vi "NPSV test.vi"() -> ()   [LabVIEW 2017]
uses:
  <vilib>/WPC Systems Ltd/GECO Driver/Lib/GECOMotion/GECOMotion/_typedefine/Axis Select.ctl
  <vilib>/WPC Systems Ltd/GECO Driver/Lib/GECOMotion/GECOMotion/GECO Motion.lvclass
  <vilib>/WPC Systems Ltd/GECO Driver/Lib/GECOBase/GECO_Driver Class/Motion/_typedefine/GECO_ActiveHighLow.ctl
  <vilib>/WPC Systems Ltd/GECO Driver/Lib/GECOBase/GECO_Driver Class/GECO_Driver.lvclass
  <vilib>/WPC Systems Ltd/GECO Driver/Lib/GECOBase/GECO_Driver Class/Motion/_typedefine/GECO_Motion Operation Mode.ctl
  GyroDef.ctl
  DataDef.ctl
  <vilib>/WPC Systems Ltd/GECO Driver/Lib/GECOBase/GECO_Driver Class/GECO_SlotName.ctl
  <vilib>/WPC Systems Ltd/GECO Driver/Lib/GECOBase/GECO_Driver Class/Motion/_typedefine/GECO_Stepper Output Configuration.ctl
  <vilib>/NI/Modbus Library/API/Modbus API.lvclass
  <vilib>/addons/control/pid/NI_PID_pid.lvlib
  <vilib>/addons/control/pid/pid.llb/PID (DBL).vi
  <vilib>/NI/Modbus Library/API/Wrapper/API Main.lvlib
  <vilib>/NI/Modbus Library/API/Wrapper/Create TCP Slave.vi
  <vilib>/WPC Systems Ltd/GECO Driver/GECODriver/GECO_Initialize_PC/Initialize VIs/Initialize_GECOUno_4HX.vi
  <vilib>/NI/Modbus Library/API/Slave/Modbus Slave.lvclass
  C:/Program Files (x86)/National Instruments/LabVIEW 2019/vi.lib/NI/Modbus Library/API/Modbus API.lvclass
panel:
  out "Axis 1":T1
  out "Axis 2":T1
  out "Axis 3":T1
  out "Program Period":u32
  in  "Main Setting Tab":T2(tab)
  in  "PID gains setting Tab":enum32{"Axis 1", "Axis 2", "Axis 3"}(tab)
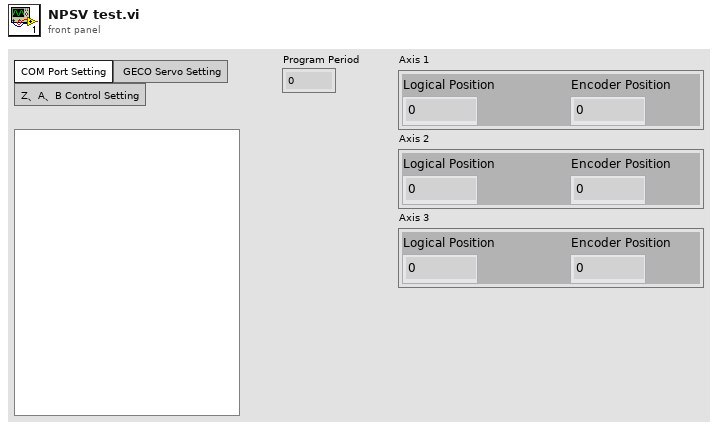
[diagram p1: front panel]
types:
  T1 = cluster{"Encoder Position":i32, "Logical Position":i32}
  T2 = enum32{"COM Port Setting", " GECO Servo Setting", "Z、A、B Control Setting"}
  T3 = typedef "DataDef.ctl" = cluster{"address starting":u16, "狀態":enum16{"初始化", "讀取", "寫入", "停止"}, "理想角度":cluster{"A":dbl, "B":dbl}, "register values":i16[], "Modbus COM":refnum<class "Modbus API.lvclass">, "TCP slave port":u16, " baud rate":u32, "Byte bits":u16, "ServoButtonControl":cluster{"三軸同退":bool, "三軸同進":bool, "三軸後退":bool, "三軸前進":bool, "二軸後退":bool, "二軸前進":bool, "一軸後退":bool, "一軸前進":bool}, "Serial Number":string, "GECO_Driver out":refnum<class "GECO_Driver.lvclass">, "number of inputs":u16, "ServoSetting":cluster{"Axis Select":T4, "Stepper Output Configuration":T5, "Motion Operation Mode":T6, "Motion Controller Slot":T7, "Singel Axis Move Paramters":cluster{"Motion Operation Mode":T6, "Target Position (0)":i32, "Velocity (10000)":i32, "Acceleration (100000)":u32, "Deacceleration (100000)":u32}, "Reverse":cluster{"Reverse Enable":bool, "Reverse Polarity":T8}, "Forward":cluster{"Forward Enable":bool, "Forward Polarity":T8}}, "GECO Motion out":refnum<class "GECO Motion.lvclass">, "Servo on":bool, "Axis 1 Position":cluster{"Encoder Position":i32, "Logical Position":i32}, "Axis 2 Position":cluster{"Encoder Position":i32, "Logical Position":i32}, "Axis 3 Position":cluster{"Encoder Position":i32, "Logical Position":i32}, "PIDSetting":cluster{"Z":i32, "A":i32, "B":i32, "Move Setting":T9, "Axis Pulse":dbl, "Axis Length":dbl, "PID gains ":cluster{"proportional gain (Kc)":dbl, "integral time (Ti, min)":dbl, "derivative time (Td, min)":dbl}}, "resource name":tag, "Save Path":refnum<file>}
  T4 = typedef "GECO Motion.lvclass/Axis Select.ctl" = enum16{"Axis 1", "Axis 2", "Axis 3", "Axis 4"}
  T5 = typedef "GECO_Driver.lvclass/GECO_Stepper Output Configuration.ctl" = enum16{"Step/Dir(One Pulse)", "CW/CCW(Two Pulse)"}
  T6 = typedef "GECO_Driver.lvclass/GECO_Motion Operation Mode.ctl" = enum16{"Absolute Position", "Relative Position", "Velocity"}
  T7 = typedef "GECO_Driver.lvclass/GECO_SlotName.ctl" = enum16{"C1", "C2", "C3", "C4"}
  T8 = typedef "GECO_Driver.lvclass/GECO_ActiveHighLow.ctl" = enum16{"Active High", "Active Low"}
  T9 = typedef "­y¸ñ.ctl" = u16
  T10 = typedef "GyroDef.ctl" = cluster{"Byte bits":u16, "baud rate":u32, "實際角度":cluster{"A":dbl, "B":dbl}, "COM Port":refnum<visa-resource-name>, "Save Path":refnum<file>}
  T11 = cluster{"Motion Operation Mode":T6, "Target Position (0)":i32, "Velocity (10000)":i32, "Acceleration (100000)":u32, "Deacceleration (100000)":u32}
  T12 = cluster{"Forward Enable":bool, "Forward Polarity":T8}
  T13 = cluster{"Reverse Enable":bool, "Reverse Polarity":T8}
  T14 = cluster{"三軸同退":bool, "三軸同進":bool, "三軸後退":bool, "三軸前進":bool, "二軸後退":bool, "二軸前進":bool, "一軸後退":bool, "一軸前進":bool, "Reset Encoder Position":bool, "AlarmReset":bool}[]
  T15 = cluster{"三軸同退":bool, "三軸同進":bool, "三軸後退":bool, "三軸前進":bool, "二軸後退":bool, "二軸前進":bool, "一軸後退":bool, "一軸前進":bool, "Reset Encoder Position":bool, "AlarmReset":bool}
  T16 = enum16{"open", "replace", "create", "open or create", "replace or create", "replace or create with confirmation"}
  T17 = cluster{"Logical Position":i32, "Encoder Position":i32}
  T18 = enum16{"Step/Dir(One Pulse)", "CW/CCW(Two Pulse)"}
  T19 = enum16{"Absolute Position", "Relative Position", "Velocity"}
  T20 = cluster{"proportional gain (Kc)":dbl, "integral time (Ti, min)":dbl, "derivative time (Td, min)":dbl}
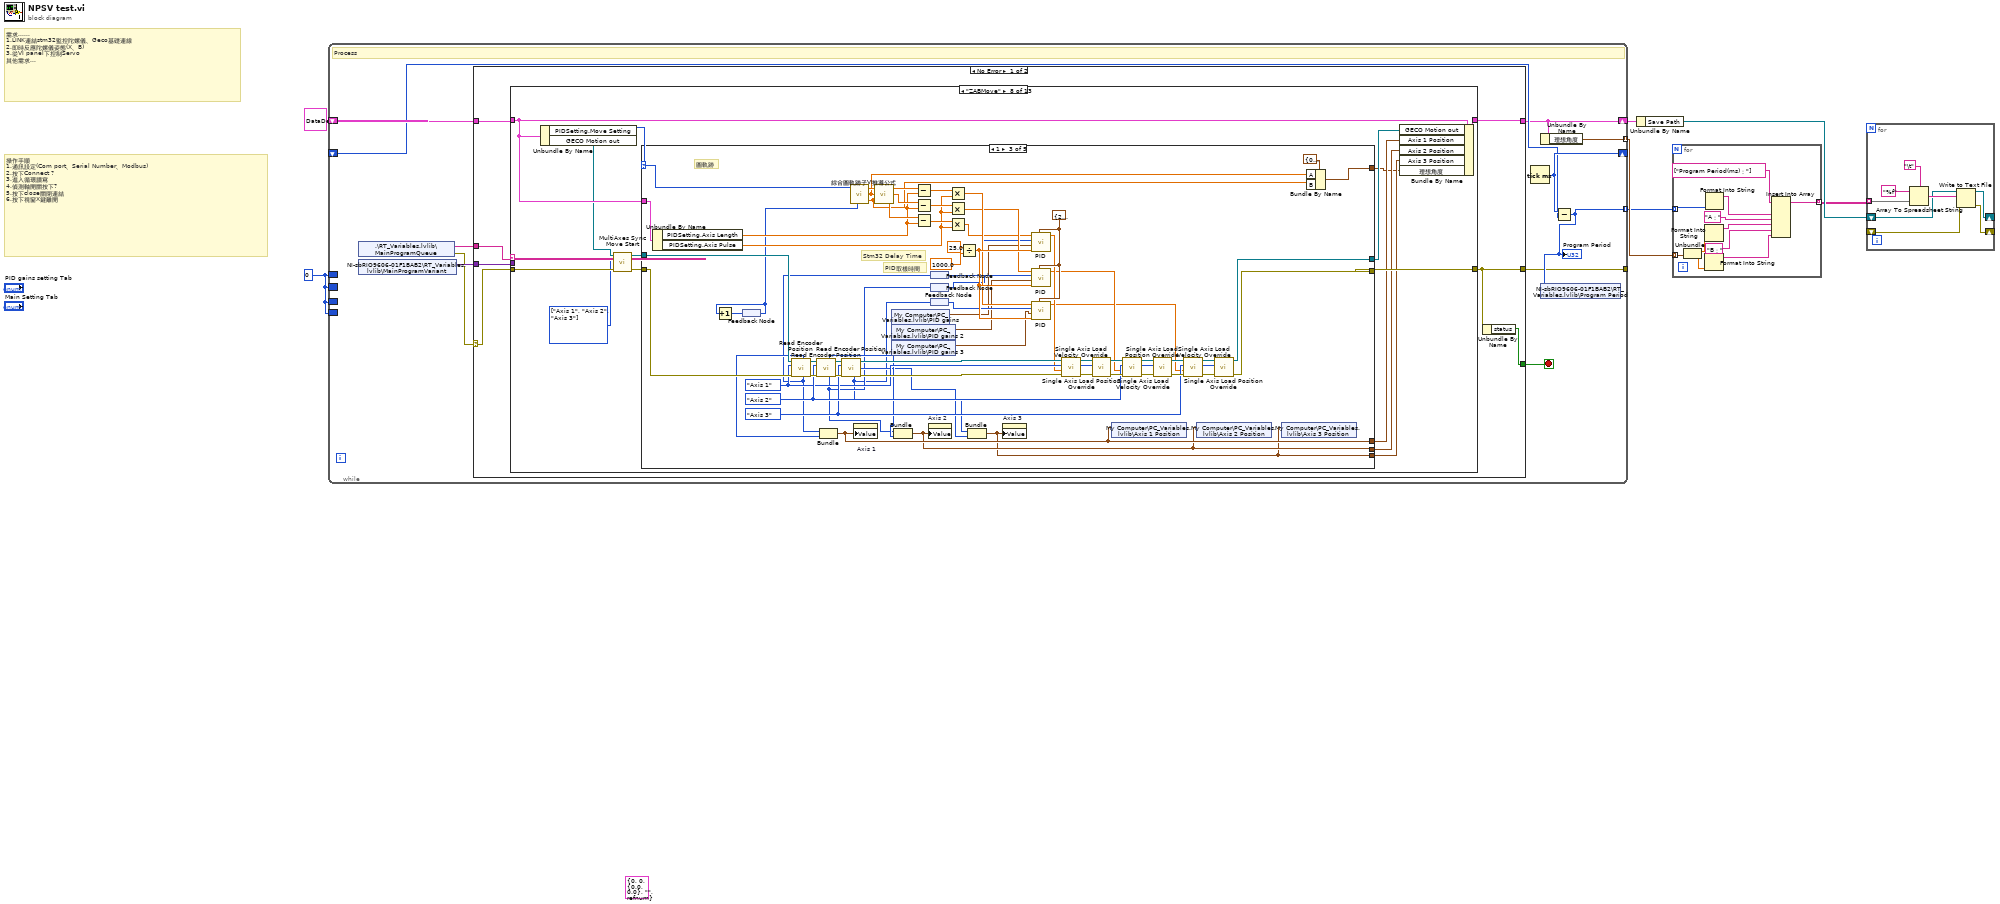
[diagram p0: block diagram]
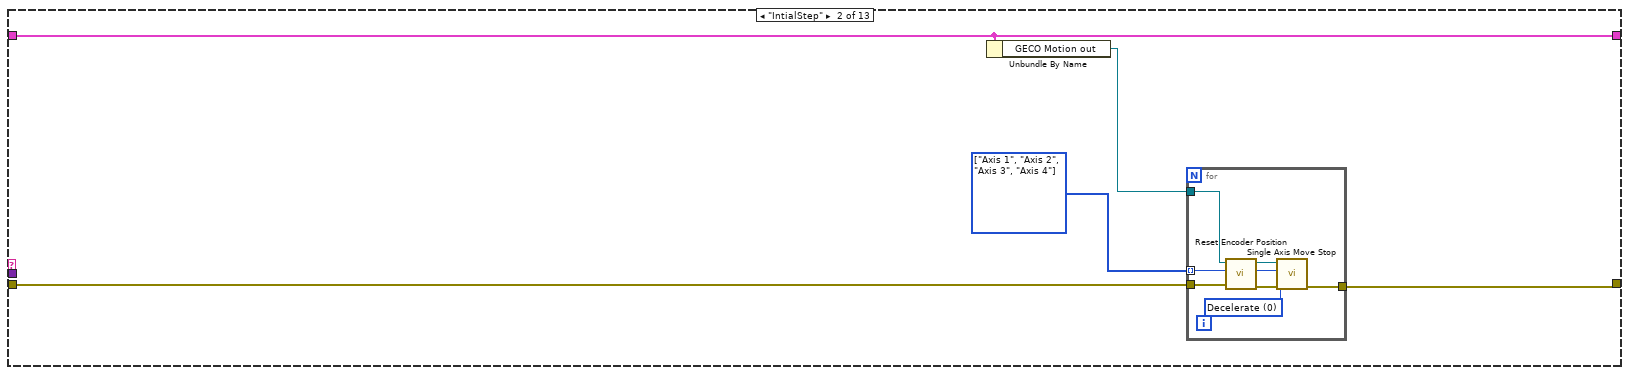
[diagram p3: hidden frame]
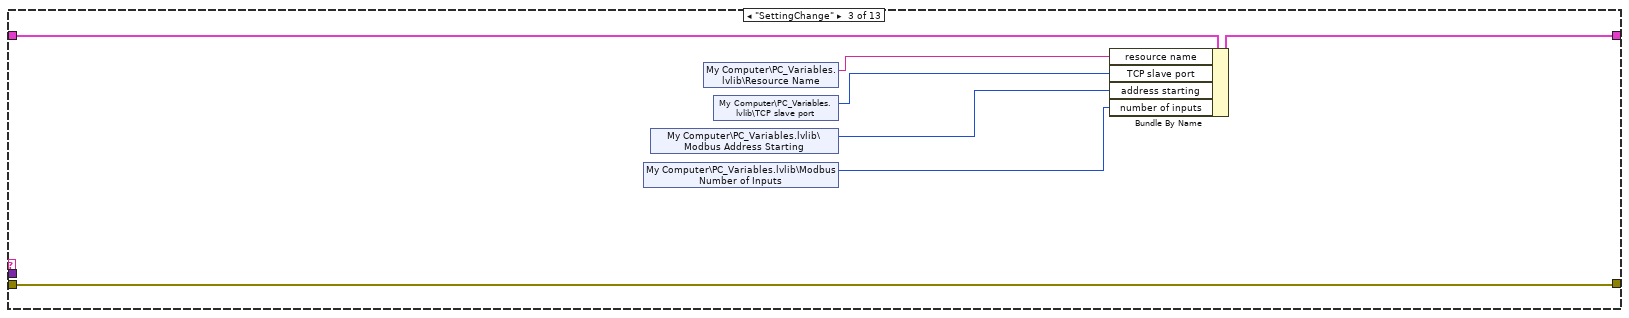
[diagram p4: hidden frame]
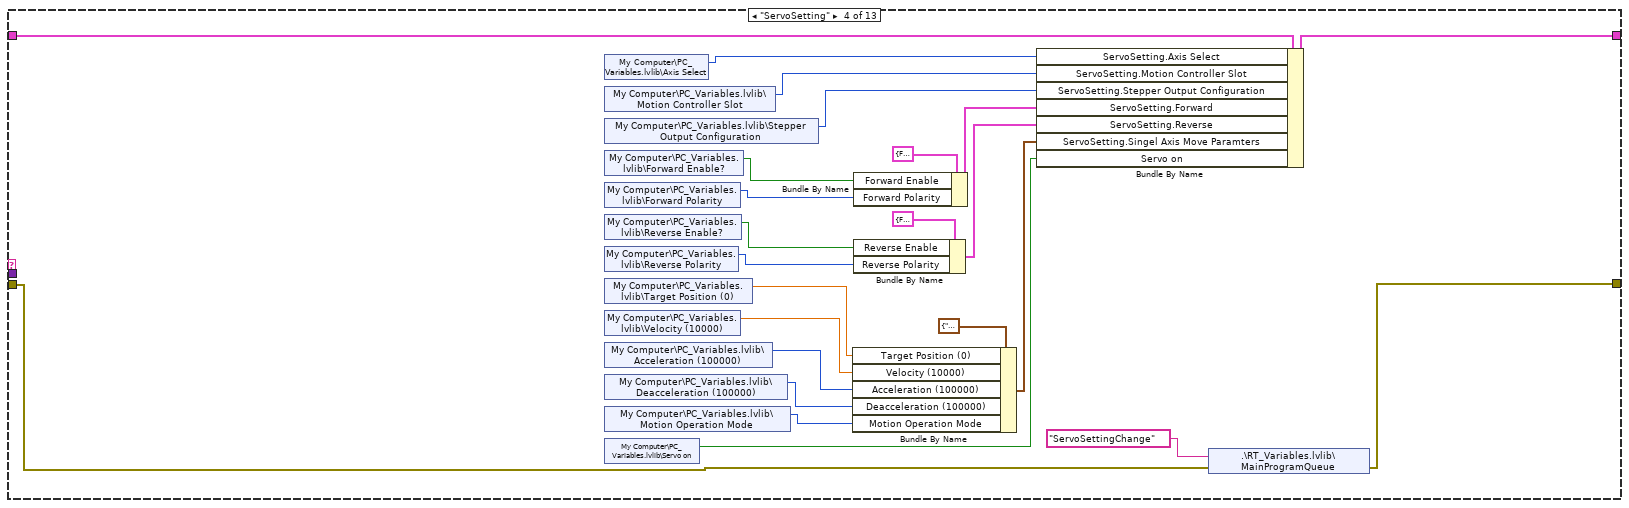
[diagram p5: hidden frame]
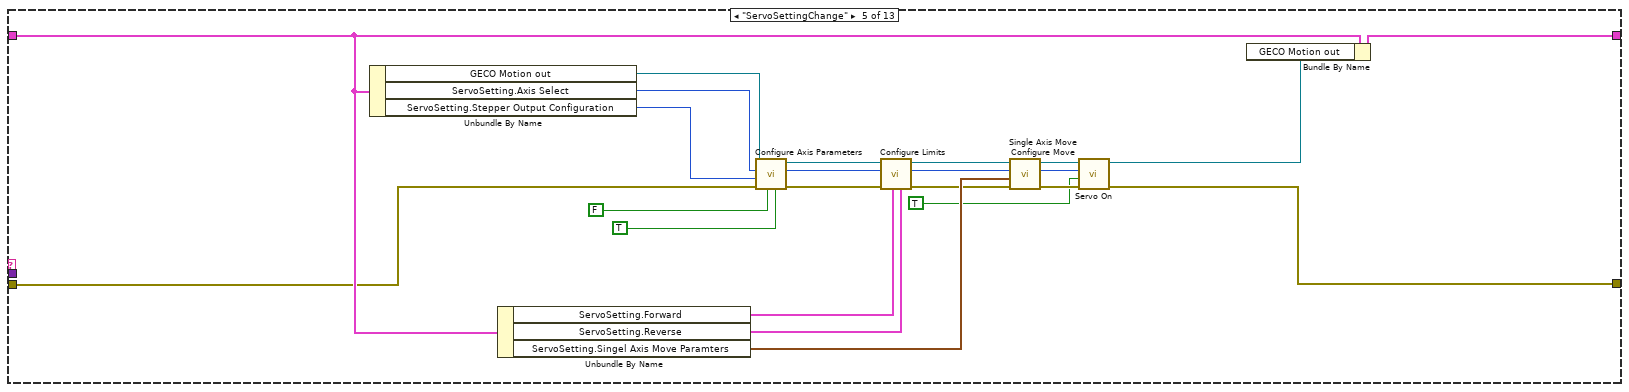
[diagram p6: hidden frame]
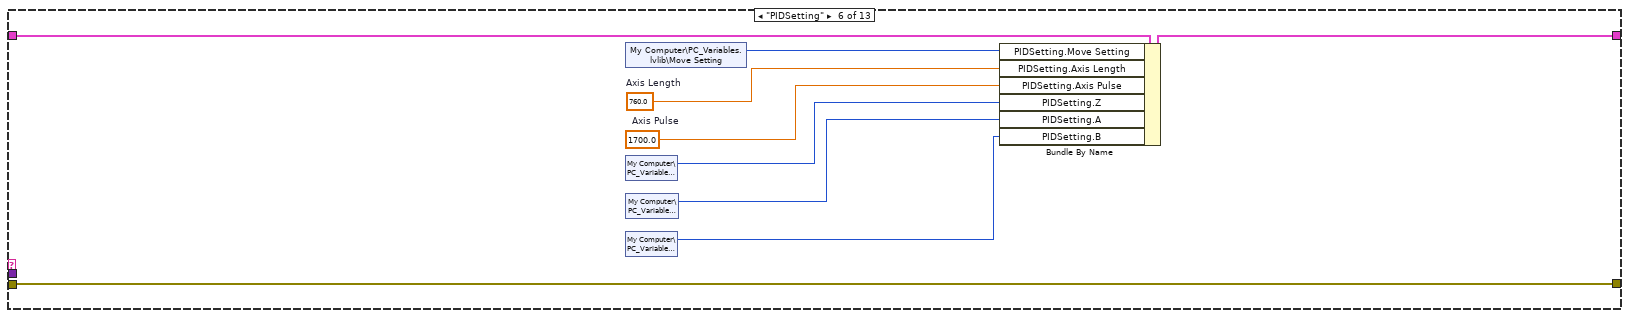
[diagram p7: hidden frame]
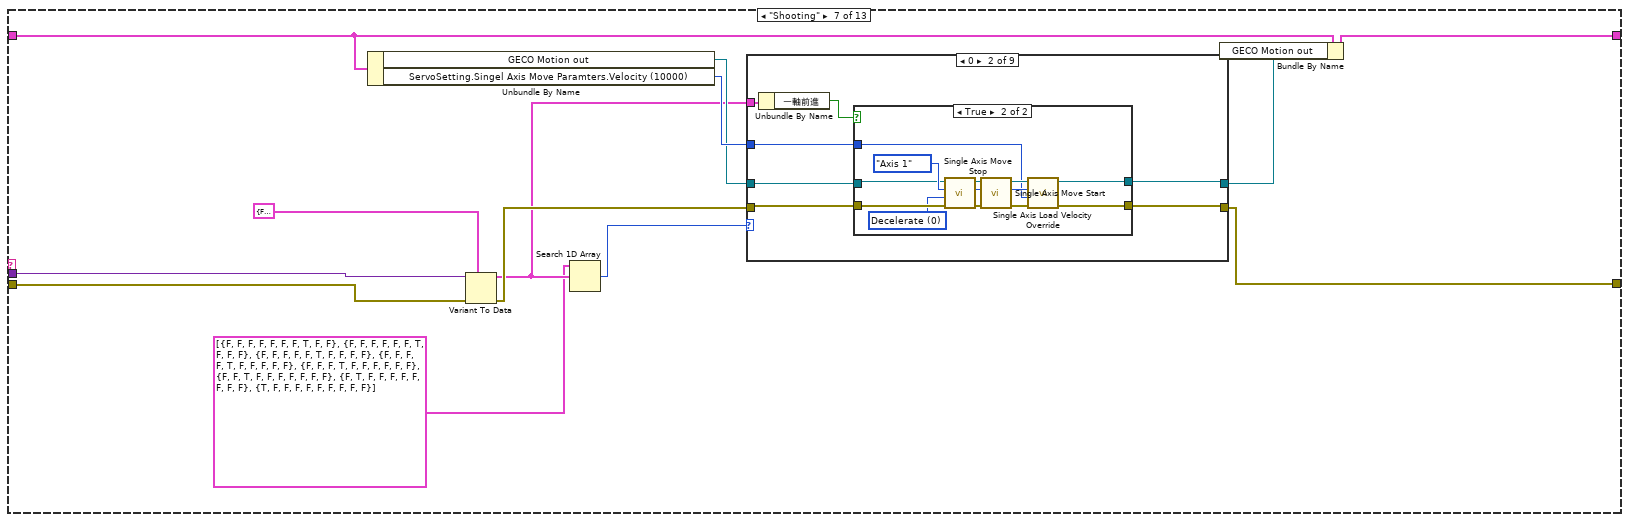
[diagram p8: hidden frame]
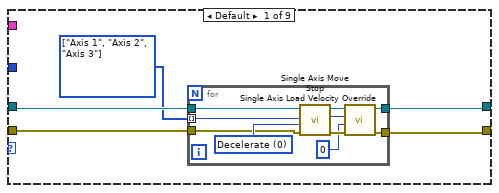
[diagram p9: hidden frame]
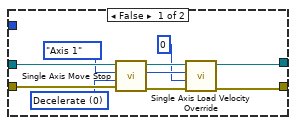
[diagram p10: hidden frame]
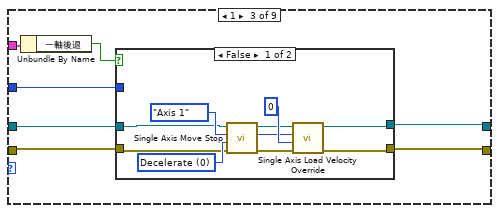
[diagram p11: hidden frame]
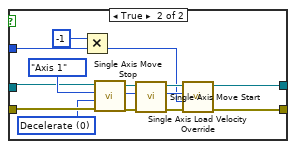
[diagram p12: hidden frame]
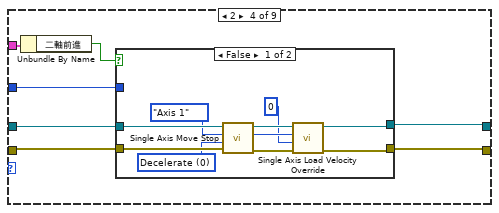
[diagram p13: hidden frame]
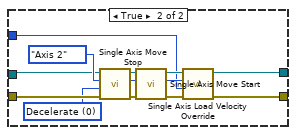
[diagram p14: hidden frame]
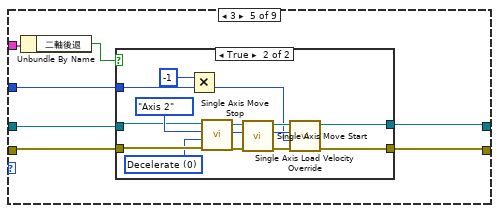
[diagram p15: hidden frame]
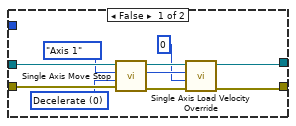
[diagram p16: hidden frame]
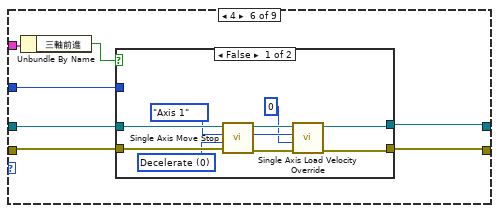
[diagram p17: hidden frame]
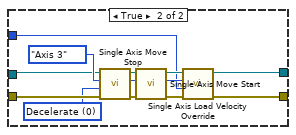
[diagram p18: hidden frame]
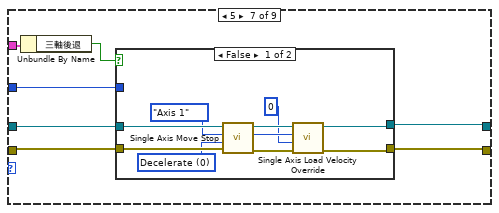
[diagram p19: hidden frame]
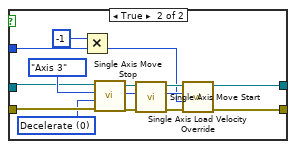
[diagram p20: hidden frame]
diagram:
  w6 = 0
  (unwired) T10 {"Byte bits"=0, "baud rate"=0, "實際角度"={"A"=0.0, "B"=0.0}, "COM Port"="", "Save Path"=refnum}
  # "操作手順\n1.通訊設定(Com port、Serial Number、Modbus)\n2.按下Connect ?\n3.進入循環讀寫\n4.偵測軸開關按下?\n5.按下close關閉連結\n6.按下視窗X鍵離開"
  # "需求......\n1.LINK連結stm32監控陀螺儀、Geco基礎連線\n2.即時反應陀螺儀姿態(X、B)\n3.從VI panel下控制Servo\n其他需求..."
  n1 = while {
    shift-right: [w14] -> w3
    shift-left: T3 {"address starting"=0, "狀態"=enum."初始化", "理想角度"={"A"=0.0, "B"=0.0}, "register values"=[], "Modbus COM"=refnum, "TCP slave port"=1, " baud rate"=0, "Byte bits"=0, "ServoButtonControl"={"三軸同退"=FALSE, "三軸同進"=FALSE, "三軸後退"=FALSE, "三軸前進"=FALSE, "二軸後退"=FALSE, "二軸前進"=FALSE, "一軸後退"=FALSE, "一軸前進"=FALSE}, "Serial Number"="", "GECO_Driver out"=refnum, "number of inputs"=0, "ServoSetting"={"Axis Select"=enum."Axis 1", "Stepper Output Configuration"=enum."Step/Dir(One Pulse)", "Motion Operation Mode"=enum."Absolute Position", "Motion Controller Slot"=enum."C1", "Singel Axis Move Paramters"={"Motion Operation Mode"=enum."Velocity", "Target Position (0)"=10000, "Velocity (10000)"=1, "Acceleration (100000)"=100000, "Deacceleration (100000)"=1}, "Reverse"={"Reverse Enable"=FALSE, "Reverse Polarity"=enum."Active Low"}, "Forward"={"Forward Enable"=FALSE, "Forward Polarity"=enum."Active Low"}}, "GECO Motion out"=refnum, "Servo on"=FALSE, "Axis 1 Position"={"Encoder Position"=0, "Logical Position"=0}, "Axis 2 Position"={"Encoder Position"=0, "Logical Position"=0}, "Axis 3 Position"={"Encoder Position"=0, "Logical Position"=0}, "PIDSetting"={"Z"=10000, "A"=10000, "B"=10000, "Move Setting"=1, "Axis Pulse"=10000.0, "Axis Length"=10000.0, "PID gains "={"proportional gain (Kc)"=1.0, "integral time (Ti, min)"=0.01, "derivative time (Td, min)"=0.0}}, "resource name"="", "Save Path"=refnum} -> [w17]
    shift-right: [w16] -> _
    shift-left: _ -> [w15]
    border: w6 -> [_]
    border: w6 -> [_]
    border: w6 -> [_]
    border: w6 -> [_]
    tunnel: [w13] -> w5 mode=indexing
    tunnel: [w12] -> w4 mode=indexing
    tunnel: [w11] -> _
    stop <- w18 stop-if-true
    # "Process"
    n2 = shared-variable ".\\RT_Variables.lvlib\\MainProgramQueue"() -> (w9:string, error out=w8:errorcluster)  [unwired: 1 in]
    n3 = shared-variable "NI-sbRIO9606-01F1BAB2\\RT_Variables.lvlib\\MainProgramVariant"() -> (w10:variant)  [unwired: 1 in, 1 out]
    n4 = case shown="No Error" w8 {
      selector: w8 -> [w23 w629]
      tunnel: [w22 TRUE] -> w18
      tunnel: [w25 w630] -> w14
      tunnel: w17 -> [w24 w630]
      tunnel: [w21 w629] -> w11
      tunnel: w10 -> [w20 _]
      tunnel: w9 -> [w19 _]
      frame No Error {
        n5 = case shown="\"ZABMove\"" w19 {
          tunnel: [w27 w29 w46 w70 w94 w102 w114 w404 w538 w554 w587 w609 w620] -> w25
          tunnel: w24 -> [w27 w29 w47 w71 w93 w103 w108 w406 w541 w557 w588 w611 w620]
          tunnel: w23 -> [w26 w28 w43 w49 w86 w95 w116 w397 w540 w556 w570 w613 w618]
          tunnel: [w26 w32 w43 w50 w80 w95 w107 w405 w536 w552 w582 w612 w619] -> w21
          tunnel: w20 -> [_ _ _ _ _ _ w115 _ _ _ _ _ _]
          frame Default {
          }
          frame "IntialStep" {
            w30 = T4[] [enum."Axis 1", enum."Axis 2", enum."Axis 3", enum."Axis 4"] items=["Axis 1", "Axis 2", "Axis 3", "Axis 4"]
            n6 = Unbundle By Name(w29) -> ("GECO Motion out"=w31:refnum<class "GECO Motion.lvclass">)
            n7 = for {
              tunnel: [w35] -> w32
              tunnel: w31 -> [w40]
              tunnel: w30 -> [w39] mode=indexing
              tunnel: w28 -> [w33]
              w34 = u16 0 items=["Decelerate", "Halt"] ("Motion Stop Type")
              n8 = call <vilib>:"Reset Encoder Position.vi"("error in (no error)"=w33, "Axis Select"=w39, "GECO Motion in"=w40) -> ("error out"=w38:errorcluster, "Axis Select out"=w37:T4, "GECO Motion out"=w36:refnum<class "GECO Motion.lvclass">)  [unwired: 6 in]
              n9 = call <vilib>:"Single Axis Move Stop.vi"("error in (no error)"=w38, "Motion Stop Type"=w34, "Axis Select"=w37, "GECO Motion in"=w36) -> ("error out"=w35:errorcluster)  [unwired: 5 in, 2 out]
            }
          }
          frame "SettingChange" {
            n10 = shared-variable "My Computer\\PC_Variables.lvlib\\Modbus Number of Inputs"() -> (w42:u32)  [unwired: 1 in, 1 out]
            n11 = shared-variable "My Computer\\PC_Variables.lvlib\\Modbus Address Starting"() -> (w44:u32)  [unwired: 1 in, 1 out]
            n12 = shared-variable "My Computer\\PC_Variables.lvlib\\Resource Name"() -> (w41:tag)  [unwired: 1 in, 1 out]
            n13 = shared-variable "My Computer\\PC_Variables.lvlib\\TCP slave port"() -> (w45:u32)  [unwired: 1 in, 1 out]
            n14 = Bundle By Name(cluster=w47, "resource name"=w41, "TCP slave port"=w45, "address starting"=w44, "number of inputs"=w42) -> (w46:T3)
          }
          frame "ServoSetting" {
            n15 = shared-variable "My Computer\\PC_Variables.lvlib\\Axis Select"() -> (w69:enum16{"Axis 1", "Axis 2", "Axis 3", "Axis 4"})  [unwired: 1 in, 1 out]
            n16 = shared-variable "My Computer\\PC_Variables.lvlib\\Motion Controller Slot"() -> (w68:enum16{"C1", "C2", "C3", "C4"})  [unwired: 1 in, 1 out]
            n17 = shared-variable "My Computer\\PC_Variables.lvlib\\Stepper Output Configuration"() -> (w67:T18)  [unwired: 1 in, 1 out]
            n18 = shared-variable "My Computer\\PC_Variables.lvlib\\Forward Enable?"() -> (w55:bool)  [unwired: 1 in, 1 out]
            n19 = shared-variable "My Computer\\PC_Variables.lvlib\\Forward Polarity"() -> (w56:enum16{"Active High", "Active Low"})  [unwired: 1 in, 1 out]
            n20 = shared-variable "My Computer\\PC_Variables.lvlib\\Reverse Enable?"() -> (w58:bool)  [unwired: 1 in, 1 out]
            n21 = shared-variable "My Computer\\PC_Variables.lvlib\\Reverse Polarity"() -> (w57:enum16{"Active High", "Active Low"})  [unwired: 1 in, 1 out]
            n22 = shared-variable "My Computer\\PC_Variables.lvlib\\Target Position (0)"() -> (w59:dbl)  [unwired: 1 in, 1 out]
            n23 = shared-variable "My Computer\\PC_Variables.lvlib\\Velocity (10000)"() -> (w60:dbl)  [unwired: 1 in, 1 out]
            n24 = shared-variable "My Computer\\PC_Variables.lvlib\\Acceleration (100000)"() -> (w61:u32)  [unwired: 1 in, 1 out]
            n25 = shared-variable "My Computer\\PC_Variables.lvlib\\Deacceleration (100000)"() -> (w62:u32)  [unwired: 1 in, 1 out]
            n26 = shared-variable "My Computer\\PC_Variables.lvlib\\Motion Operation Mode"() -> (w63:T19)  [unwired: 1 in, 1 out]
            n27 = shared-variable "My Computer\\PC_Variables.lvlib\\Servo on"() -> (w51:bool)  [unwired: 1 in, 1 out]
            n28 = Bundle By Name(cluster=T11 {"Motion Operation Mode"=enum."Absolute Position", "Target Position (0)"=0, "Velocity (10000)"=10000, "Acceleration (100000)"=100000, "Deacceleration (100000)"=100000} ("Singel Axis Move Paramters"), "Target Position (0)"=w59, "Velocity (10000)"=w60, "Acceleration (100000)"=w61, "Deacceleration (100000)"=w62, "Motion Operation Mode"=w63) -> (w52:T11)
            n29 = Bundle By Name(cluster=T12 {"Forward Enable"=FALSE, "Forward Polarity"=enum."Active Low"} ("Forward"), "Forward Enable"=w55, "Forward Polarity"=w56) -> (w54:T12)
            n30 = Bundle By Name(cluster=T13 {"Reverse Enable"=FALSE, "Reverse Polarity"=enum."Active Low"} ("Reverse"), "Reverse Enable"=w58, "Reverse Polarity"=w57) -> (w53:T13)
            n31 = Bundle By Name(cluster=w71, "ServoSetting.Axis Select"=w69, "ServoSetting.Motion Controller Slot"=w68, "ServoSetting.Stepper Output Configuration"=w67, "ServoSetting.Forward"=w54, "ServoSetting.Reverse"=w53, "ServoSetting.Singel Axis Move Paramters"=w52, "Servo on"=w51) -> (w70:T3)
            n32 = shared-variable ".\\RT_Variables.lvlib\\MainProgramQueue"("ServoSettingChange", error in=w49) -> (error out=w50:errorcluster)
          }
          frame "ServoSettingChange" {
            n33 = Unbundle By Name(w93) -> ("GECO Motion out"=w87:refnum<class "GECO Motion.lvclass">, "ServoSetting.Axis Select"=w91:T4, "ServoSetting.Stepper Output Configuration"=w90:T5)
            n34 = Unbundle By Name(w93) -> ("ServoSetting.Forward"=w73:T12, "ServoSetting.Reverse"=w72:T13, "ServoSetting.Singel Axis Move Paramters"=w92:T11)
            n35 = call <vilib>:"Configure Axis Parameters.vi"("Reverse Encoder Direction?"=TRUE, "Reverse Axis Direction?"=FALSE, "error in (no error)"=w86, "Stepper Output Configuration"=w90, "Axis Select"=w91, "GECO Motion in"=w87) -> ("error out"=w77:errorcluster, "Axis Select out"=w79:T4, "GECO Motion out"=w78:refnum<class "GECO Motion.lvclass">)  [unwired: 3 in]
            n36 = call <vilib>:"Configure Limits.vi"("Reverse"=w72, "Forward"=w73, "error in (no error)"=w77, "Axis Select"=w79, "GECO Motion in"=w78) -> ("error out"=w74:errorcluster, "Axis Select out"=w75:T4, "GECO Motion out"=w76:refnum<class "GECO Motion.lvclass">)  [unwired: 4 in]
            n37 = call <vilib>:"Single Axis Move Configure Move.vi"("error in (no error)"=w74, "Singel Axis Move Paramters"=w92, "Axis Select"=w75, "GECO Motion in"=w76) -> ("error out"=w83:errorcluster, "Axis Select out"=w84:T4, "GECO Motion out"=w85:refnum<class "GECO Motion.lvclass">)  [unwired: 5 in]
            n38 = call <vilib>:"Servo On.vi"("error in (no error)"=w83, "Servo On"=TRUE, "Axis Select"=w84, "GECO Motion in"=w85) -> ("error out"=w80:errorcluster, "GECO Motion out"=w81:refnum<class "GECO Motion.lvclass">)  [unwired: 5 in, 1 out]
            n39 = Bundle By Name(cluster=w93, "GECO Motion out"=w81) -> (w94:T3)
          }
          frame "PIDSetting" {
            w99 = 1700.0  # Axis Pulse
            w100 = 760.0  # Axis Length
            n40 = shared-variable "My Computer\\PC_Variables.lvlib\\Move Setting"() -> (w101:u16)  [unwired: 1 in, 1 out]
            n41 = shared-variable "My Computer\\PC_Variables.lvlib\\Z"() -> (w98:i32)  [unwired: 1 in, 1 out]
            n42 = shared-variable "My Computer\\PC_Variables.lvlib\\A"() -> (w97:i32)  [unwired: 1 in, 1 out]
            n43 = shared-variable "My Computer\\PC_Variables.lvlib\\B"() -> (w96:i32)  [unwired: 1 in, 1 out]
            n44 = Bundle By Name(cluster=w103, "PIDSetting.Move Setting"=w101, "PIDSetting.Axis Length"=w100, "PIDSetting.Axis Pulse"=w99, "PIDSetting.Z"=w98, "PIDSetting.A"=w97, "PIDSetting.B"=w96) -> (w102:T3)
          }
          frame "Shooting" {
            n45 = Unbundle By Name(w108) -> ("GECO Motion out"=w110:refnum<class "GECO Motion.lvclass">, "ServoSetting.Singel Axis Move Paramters.Velocity (10000)"=w111:i32)
            n46 = Variant To Data(error in=w116, type=T15 {"三軸同退"=FALSE, "三軸同進"=FALSE, "三軸後退"=FALSE, "三軸前進"=FALSE, "二軸後退"=FALSE, "二軸前進"=FALSE, "一軸後退"=FALSE, "一軸前進"=FALSE, "Reset Encoder Position"=FALSE, "AlarmReset"=FALSE} ("ServoButtonControl"), Variant=w115) -> (data=w106:T15, error out=w112:errorcluster)
            n47 = Search 1D Array(1D array=T14 [{"三軸同退"=FALSE, "三軸同進"=FALSE, "三軸後退"=FALSE, "三軸前進"=FALSE, "二軸後退"=FALSE, "二軸前進"=FALSE, "一軸後退"=FALSE, "一軸前進"=TRUE, "Reset Encoder Position"=FALSE, "AlarmReset"=FALSE}, {"三軸同退"=FALSE, "三軸同進"=FALSE, "三軸後退"=FALSE, "三軸前進"=FALSE, "二軸後退"=FALSE, "二軸前進"=FALSE, "一軸後退"=TRUE, "一軸前進"=FALSE, "Reset Encoder Position"=FALSE, "AlarmReset"=FALSE}, {"三軸同退"=FALSE, "三軸同進"=FALSE, "三軸後退"=FALSE, "三軸前進"=FALSE, "二軸後退"=FALSE, "二軸前進"=TRUE, "一軸後退"=FALSE, "一軸前進"=FALSE, "Reset Encoder Position"=FALSE, "AlarmReset"=FALSE}, {"三軸同退"=FALSE, "三軸同進"=FALSE, "三軸後退"=FALSE, "三軸前進"=FALSE, "二軸後退"=TRUE, "二軸前進"=FALSE, "一軸後退"=FALSE, "一軸前進"=FALSE, "Reset Encoder Position"=FALSE, "AlarmReset"=FALSE}, {"三軸同退"=FALSE, "三軸同進"=FALSE, "三軸後退"=FALSE, "三軸前進"=TRUE, "二軸後退"=FALSE, "二軸前進"=FALSE, "一軸後退"=FALSE, "一軸前進"=FALSE, "Reset Encoder Position"=FALSE, "AlarmReset"=FALSE}, {"三軸同退"=FALSE, "三軸同進"=FALSE, "三軸後退"=TRUE, "三軸前進"=FALSE, "二軸後退"=FALSE, "二軸前進"=FALSE, "一軸後退"=FALSE, "一軸前進"=FALSE, "Reset Encoder Position"=FALSE, "AlarmReset"=FALSE}, {"三軸同退"=FALSE, "三軸同進"=TRUE, "三軸後退"=FALSE, "三軸前進"=FALSE, "二軸後退"=FALSE, "二軸前進"=FALSE, "一軸後退"=FALSE, "一軸前進"=FALSE, "Reset Encoder Position"=FALSE, "AlarmReset"=FALSE}, {"三軸同退"=TRUE, "三軸同進"=FALSE, "三軸後退"=FALSE, "三軸前進"=FALSE, "二軸後退"=FALSE, "二軸前進"=FALSE, "一軸後退"=FALSE, "一軸前進"=FALSE, "Reset Encoder Position"=FALSE, "AlarmReset"=FALSE}], element=w106) -> (index of element=w113:i32)  [unwired: 1 in]
            n48 = case shown="0" w113 {
              tunnel: w112 -> [w120 w137 w167 w199 w229 w261 w291 w323 w360]
              tunnel: w111 -> [_ w136 w166 w198 w228 w260 w290 w322 w359]
              tunnel: w110 -> [w121 w138 w168 w200 w230 w262 w292 w324 w361]
              tunnel: [w118 w135 w165 w197 w227 w259 w289 w321 w358] -> w109
              tunnel: [w117 w134 w164 w196 w226 w258 w288 w320 w357] -> w107
              tunnel: w106 -> [_ w133 w163 w195 w225 w257 w287 w319 w356]
              frame Default {
                w119 = T4[] [enum."Axis 1", enum."Axis 2", enum."Axis 3"] items=["Axis 1", "Axis 2", "Axis 3", "Axis 4"] ("Start Axes Select")
                n49 = for {
                  tunnel: w120 -> [w130]
                  tunnel: w121 -> [w129]
                  tunnel: w119 -> [w128] mode=indexing
                  tunnel: [w123] -> w118
                  tunnel: [w124] -> w117
                  w131 = u16 0 items=["Decelerate", "Halt"] ("Motion Stop Type")
                  n50 = call <vilib>:"Single Axis Move Stop.vi"("error in (no error)"=w130, "Motion Stop Type"=w131, "Axis Select"=w128, "GECO Motion in"=w129) -> ("error out"=w126:errorcluster, "Axis Select out"=w125:T4, "GECO Motion out"=w127:refnum<class "GECO Motion.lvclass">)  [unwired: 5 in]
                  n51 = call <vilib>:"Single Axis Load Velocity Override.vi"("error in (no error)"=w126, "Override Velosity Value"=0, "Axis Select"=w125, "GECO Motion in"=w127) -> ("error out"=w124:errorcluster, "GECO Motion out"=w123:refnum<class "GECO Motion.lvclass">)  [unwired: 5 in, 1 out]
                }
              }
              frame 0 {
                n52 = Unbundle By Name(w133) -> ("一軸前進"=w132:bool)
                n53 = case shown="True" w132 {
                  tunnel: w138 -> [w148 w154]
                  tunnel: w137 -> [w147 w153]
                  tunnel: w136 -> [_ w158]
                  tunnel: [w139 w157] -> w135
                  tunnel: [w140 w156] -> w134
                  frame False {
                    w146 = u16 0 items=["Decelerate", "Halt"] ("Motion Stop Type")
                    n54 = call <vilib>:"Single Axis Move Stop.vi"("error in (no error)"=w147, "Motion Stop Type"=w146, "Axis Select"=Axis_Select."Axis 1", "GECO Motion in"=w148) -> ("error out"=w143:errorcluster, "Axis Select out"=w142:T4, "GECO Motion out"=w144:refnum<class "GECO Motion.lvclass">)  [unwired: 5 in]
                    n55 = call <vilib>:"Single Axis Load Velocity Override.vi"("error in (no error)"=w143, "Override Velosity Value"=0, "Axis Select"=w142, "GECO Motion in"=w144) -> ("error out"=w140:errorcluster, "GECO Motion out"=w139:refnum<class "GECO Motion.lvclass">)  [unwired: 5 in, 1 out]
                  }
                  frame True {
                    w152 = u16 0 items=["Decelerate", "Halt"] ("Motion Stop Type")
                    n56 = call <vilib>:"Single Axis Move Stop.vi"("error in (no error)"=w153, "Motion Stop Type"=w152, "Axis Select"=Axis_Select."Axis 1", "GECO Motion in"=w154) -> ("error out"=w150:errorcluster, "Axis Select out"=w149:T4, "GECO Motion out"=w151:refnum<class "GECO Motion.lvclass">)  [unwired: 5 in]
                    n57 = call <vilib>:"Single Axis Move Start.vi"("error in (no error)"=w150, "Axis Select"=w149, "GECO Motion in"=w151) -> ("error out"=w160:errorcluster, "Axis Select out"=w159:T4, "GECO Motion out"=w161:refnum<class "GECO Motion.lvclass">)  [unwired: 6 in]
                    n58 = call <vilib>:"Single Axis Load Velocity Override.vi"("error in (no error)"=w160, "Override Velosity Value"=w158, "Axis Select"=w159, "GECO Motion in"=w161) -> ("error out"=w156:errorcluster, "GECO Motion out"=w157:refnum<class "GECO Motion.lvclass">)  [unwired: 5 in, 1 out]
                  }
                }
              }
              frame 1 {
                n59 = Unbundle By Name(w163) -> ("一軸後退"=w162:bool)
                n60 = case shown="False" w162 {
                  tunnel: w168 -> [w174 w182]
                  tunnel: w167 -> [w172 w181]
                  tunnel: w166 -> [_ w190]
                  tunnel: [w176 w189] -> w165
                  tunnel: [w177 w188] -> w164
                  frame False {
                    w173 = u16 0 items=["Decelerate", "Halt"] ("Motion Stop Type")
                    n61 = call <vilib>:"Single Axis Move Stop.vi"("error in (no error)"=w172, "Motion Stop Type"=w173, "Axis Select"=Axis_Select."Axis 1", "GECO Motion in"=w174) -> ("error out"=w170:errorcluster, "Axis Select out"=w169:T4, "GECO Motion out"=w171:refnum<class "GECO Motion.lvclass">)  [unwired: 5 in]
                    n62 = call <vilib>:"Single Axis Load Velocity Override.vi"("error in (no error)"=w170, "Override Velosity Value"=0, "Axis Select"=w169, "GECO Motion in"=w171) -> ("error out"=w177:errorcluster, "GECO Motion out"=w176:refnum<class "GECO Motion.lvclass">)  [unwired: 5 in, 1 out]
                  }
                  frame True {
                    w180 = u16 0 items=["Decelerate", "Halt"] ("Motion Stop Type")
                    n63 = Multiply(x=-1, y=w190) -> (x*y=w187:i32)
                    n64 = call <vilib>:"Single Axis Move Stop.vi"("error in (no error)"=w181, "Motion Stop Type"=w180, "Axis Select"=Axis_Select."Axis 1", "GECO Motion in"=w182) -> ("error out"=w184:errorcluster, "Axis Select out"=w179:T4, "GECO Motion out"=w185:refnum<class "GECO Motion.lvclass">)  [unwired: 5 in]
                    n65 = call <vilib>:"Single Axis Move Start.vi"("error in (no error)"=w184, "Axis Select"=w179, "GECO Motion in"=w185) -> ("error out"=w192:errorcluster, "Axis Select out"=w191:T4, "GECO Motion out"=w193:refnum<class "GECO Motion.lvclass">)  [unwired: 6 in]
                    n66 = call <vilib>:"Single Axis Load Velocity Override.vi"("error in (no error)"=w192, "Override Velosity Value"=w187, "Axis Select"=w191, "GECO Motion in"=w193) -> ("error out"=w188:errorcluster, "GECO Motion out"=w189:refnum<class "GECO Motion.lvclass">)  [unwired: 5 in, 1 out]
                  }
                }
              }
              frame 2 {
                n67 = Unbundle By Name(w195) -> ("二軸前進"=w194:bool)
                n68 = case shown="False" w194 {
                  tunnel: w200 -> [w210 w216]
                  tunnel: w199 -> [w209 w215]
                  tunnel: w198 -> [_ w220]
                  tunnel: [w201 w219] -> w197
                  tunnel: [w202 w218] -> w196
                  frame False {
                    w208 = u16 0 items=["Decelerate", "Halt"] ("Motion Stop Type")
                    n69 = call <vilib>:"Single Axis Move Stop.vi"("error in (no error)"=w209, "Motion Stop Type"=w208, "Axis Select"=Axis_Select."Axis 1", "GECO Motion in"=w210) -> ("error out"=w205:errorcluster, "Axis Select out"=w204:T4, "GECO Motion out"=w206:refnum<class "GECO Motion.lvclass">)  [unwired: 5 in]
                    n70 = call <vilib>:"Single Axis Load Velocity Override.vi"("error in (no error)"=w205, "Override Velosity Value"=0, "Axis Select"=w204, "GECO Motion in"=w206) -> ("error out"=w202:errorcluster, "GECO Motion out"=w201:refnum<class "GECO Motion.lvclass">)  [unwired: 5 in, 1 out]
                  }
                  frame True {
                    w214 = u16 0 items=["Decelerate", "Halt"] ("Motion Stop Type")
                    n71 = call <vilib>:"Single Axis Move Stop.vi"("error in (no error)"=w215, "Motion Stop Type"=w214, "Axis Select"=Axis_Select."Axis 2", "GECO Motion in"=w216) -> ("error out"=w212:errorcluster, "Axis Select out"=w211:T4, "GECO Motion out"=w213:refnum<class "GECO Motion.lvclass">)  [unwired: 5 in]
                    n72 = call <vilib>:"Single Axis Move Start.vi"("error in (no error)"=w212, "Axis Select"=w211, "GECO Motion in"=w213) -> ("error out"=w222:errorcluster, "Axis Select out"=w221:T4, "GECO Motion out"=w223:refnum<class "GECO Motion.lvclass">)  [unwired: 6 in]
                    n73 = call <vilib>:"Single Axis Load Velocity Override.vi"("error in (no error)"=w222, "Override Velosity Value"=w220, "Axis Select"=w221, "GECO Motion in"=w223) -> ("error out"=w218:errorcluster, "GECO Motion out"=w219:refnum<class "GECO Motion.lvclass">)  [unwired: 5 in, 1 out]
                  }
                }
              }
              frame 3 {
                n74 = Unbundle By Name(w225) -> ("二軸後退"=w224:bool)
                n75 = case shown="True" w224 {
                  tunnel: w230 -> [w240 w244]
                  tunnel: w229 -> [w239 w243]
                  tunnel: w228 -> [_ w252]
                  tunnel: [w231 w251] -> w227
                  tunnel: [w232 w250] -> w226
                  frame False {
                    w238 = u16 0 items=["Decelerate", "Halt"] ("Motion Stop Type")
                    n76 = call <vilib>:"Single Axis Move Stop.vi"("error in (no error)"=w239, "Motion Stop Type"=w238, "Axis Select"=Axis_Select."Axis 1", "GECO Motion in"=w240) -> ("error out"=w235:errorcluster, "Axis Select out"=w234:T4, "GECO Motion out"=w236:refnum<class "GECO Motion.lvclass">)  [unwired: 5 in]
                    n77 = call <vilib>:"Single Axis Load Velocity Override.vi"("error in (no error)"=w235, "Override Velosity Value"=0, "Axis Select"=w234, "GECO Motion in"=w236) -> ("error out"=w232:errorcluster, "GECO Motion out"=w231:refnum<class "GECO Motion.lvclass">)  [unwired: 5 in, 1 out]
                  }
                  frame True {
                    w242 = u16 0 items=["Decelerate", "Halt"] ("Motion Stop Type")
                    n78 = Multiply(x=-1, y=w252) -> (x*y=w249:i32)
                    n79 = call <vilib>:"Single Axis Move Stop.vi"("error in (no error)"=w243, "Motion Stop Type"=w242, "Axis Select"=Axis_Select."Axis 2", "GECO Motion in"=w244) -> ("error out"=w246:errorcluster, "Axis Select out"=w241:T4, "GECO Motion out"=w247:refnum<class "GECO Motion.lvclass">)  [unwired: 5 in]
                    n80 = call <vilib>:"Single Axis Move Start.vi"("error in (no error)"=w246, "Axis Select"=w241, "GECO Motion in"=w247) -> ("error out"=w254:errorcluster, "Axis Select out"=w253:T4, "GECO Motion out"=w255:refnum<class "GECO Motion.lvclass">)  [unwired: 6 in]
                    n81 = call <vilib>:"Single Axis Load Velocity Override.vi"("error in (no error)"=w254, "Override Velosity Value"=w249, "Axis Select"=w253, "GECO Motion in"=w255) -> ("error out"=w250:errorcluster, "GECO Motion out"=w251:refnum<class "GECO Motion.lvclass">)  [unwired: 5 in, 1 out]
                  }
                }
              }
              frame 4 {
                n82 = Unbundle By Name(w257) -> ("三軸前進"=w256:bool)
                n83 = case shown="False" w256 {
                  tunnel: w262 -> [w272 w278]
                  tunnel: w261 -> [w271 w277]
                  tunnel: w260 -> [_ w282]
                  tunnel: [w263 w281] -> w259
                  tunnel: [w264 w280] -> w258
                  frame False {
                    w270 = u16 0 items=["Decelerate", "Halt"] ("Motion Stop Type")
                    n84 = call <vilib>:"Single Axis Move Stop.vi"("error in (no error)"=w271, "Motion Stop Type"=w270, "Axis Select"=Axis_Select."Axis 1", "GECO Motion in"=w272) -> ("error out"=w267:errorcluster, "Axis Select out"=w266:T4, "GECO Motion out"=w268:refnum<class "GECO Motion.lvclass">)  [unwired: 5 in]
                    n85 = call <vilib>:"Single Axis Load Velocity Override.vi"("error in (no error)"=w267, "Override Velosity Value"=0, "Axis Select"=w266, "GECO Motion in"=w268) -> ("error out"=w264:errorcluster, "GECO Motion out"=w263:refnum<class "GECO Motion.lvclass">)  [unwired: 5 in, 1 out]
                  }
                  frame True {
                    w276 = u16 0 items=["Decelerate", "Halt"] ("Motion Stop Type")
                    n86 = call <vilib>:"Single Axis Move Stop.vi"("error in (no error)"=w277, "Motion Stop Type"=w276, "Axis Select"=Axis_Select."Axis 3", "GECO Motion in"=w278) -> ("error out"=w274:errorcluster, "Axis Select out"=w273:T4, "GECO Motion out"=w275:refnum<class "GECO Motion.lvclass">)  [unwired: 5 in]
                    n87 = call <vilib>:"Single Axis Move Start.vi"("error in (no error)"=w274, "Axis Select"=w273, "GECO Motion in"=w275) -> ("error out"=w284:errorcluster, "Axis Select out"=w283:T4, "GECO Motion out"=w285:refnum<class "GECO Motion.lvclass">)  [unwired: 6 in]
                    n88 = call <vilib>:"Single Axis Load Velocity Override.vi"("error in (no error)"=w284, "Override Velosity Value"=w282, "Axis Select"=w283, "GECO Motion in"=w285) -> ("error out"=w280:errorcluster, "GECO Motion out"=w281:refnum<class "GECO Motion.lvclass">)  [unwired: 5 in, 1 out]
                  }
                }
              }
              frame 5 {
                n89 = Unbundle By Name(w287) -> ("三軸後退"=w286:bool)
                n90 = case shown="False" w286 {
                  tunnel: w292 -> [w302 w306]
                  tunnel: w291 -> [w301 w305]
                  tunnel: w290 -> [_ w314]
                  tunnel: [w293 w313] -> w289
                  tunnel: [w294 w312] -> w288
                  frame False {
                    w300 = u16 0 items=["Decelerate", "Halt"] ("Motion Stop Type")
                    n91 = call <vilib>:"Single Axis Move Stop.vi"("error in (no error)"=w301, "Motion Stop Type"=w300, "Axis Select"=Axis_Select."Axis 1", "GECO Motion in"=w302) -> ("error out"=w297:errorcluster, "Axis Select out"=w296:T4, "GECO Motion out"=w298:refnum<class "GECO Motion.lvclass">)  [unwired: 5 in]
                    n92 = call <vilib>:"Single Axis Load Velocity Override.vi"("error in (no error)"=w297, "Override Velosity Value"=0, "Axis Select"=w296, "GECO Motion in"=w298) -> ("error out"=w294:errorcluster, "GECO Motion out"=w293:refnum<class "GECO Motion.lvclass">)  [unwired: 5 in, 1 out]
                  }
                  frame True {
                    w304 = u16 0 items=["Decelerate", "Halt"] ("Motion Stop Type")
                    n93 = Multiply(x=-1, y=w314) -> (x*y=w311:i32)
                    n94 = call <vilib>:"Single Axis Move Stop.vi"("error in (no error)"=w305, "Motion Stop Type"=w304, "Axis Select"=Axis_Select."Axis 3", "GECO Motion in"=w306) -> ("error out"=w308:errorcluster, "Axis Select out"=w303:T4, "GECO Motion out"=w309:refnum<class "GECO Motion.lvclass">)  [unwired: 5 in]
                    n95 = call <vilib>:"Single Axis Move Start.vi"("error in (no error)"=w308, "Axis Select"=w303, "GECO Motion in"=w309) -> ("error out"=w316:errorcluster, "Axis Select out"=w315:T4, "GECO Motion out"=w317:refnum<class "GECO Motion.lvclass">)  [unwired: 6 in]
                    n96 = call <vilib>:"Single Axis Load Velocity Override.vi"("error in (no error)"=w316, "Override Velosity Value"=w311, "Axis Select"=w315, "GECO Motion in"=w317) -> ("error out"=w312:errorcluster, "GECO Motion out"=w313:refnum<class "GECO Motion.lvclass">)  [unwired: 5 in, 1 out]
                  }
                }
              }
              frame 6 {
                n97 = Unbundle By Name(w319) -> ("三軸同進"=w318:bool)
                n98 = case shown="False" w318 {
                  tunnel: w324 -> [w328 w346]
                  tunnel: w323 -> [w329 w345]
                  tunnel: w322 -> [_ w341]
                  tunnel: [w326 w354] -> w321
                  tunnel: [w325 w353] -> w320
                  frame False {
                    w327 = T4[] [enum."Axis 1", enum."Axis 2", enum."Axis 3"] items=["Axis 1", "Axis 2", "Axis 3", "Axis 4"] ("Start Axes Select")
                    n99 = for {
                      tunnel: w329 -> [w338]
                      tunnel: w328 -> [w337]
                      tunnel: w327 -> [w336] mode=indexing
                      tunnel: [w331] -> w326
                      tunnel: [w332] -> w325
                      w339 = u16 0 items=["Decelerate", "Halt"] ("Motion Stop Type")
                      n100 = call <vilib>:"Single Axis Move Stop.vi"("error in (no error)"=w338, "Motion Stop Type"=w339, "Axis Select"=w336, "GECO Motion in"=w337) -> ("error out"=w334:errorcluster, "Axis Select out"=w333:T4, "GECO Motion out"=w335:refnum<class "GECO Motion.lvclass">)  [unwired: 5 in]
                      n101 = call <vilib>:"Single Axis Load Velocity Override.vi"("error in (no error)"=w334, "Override Velosity Value"=0, "Axis Select"=w333, "GECO Motion in"=w335) -> ("error out"=w332:errorcluster, "GECO Motion out"=w331:refnum<class "GECO Motion.lvclass">)  [unwired: 5 in, 1 out]
                    }
                  }
                  frame True {
                    w342 = T4[] [enum."Axis 1", enum."Axis 2", enum."Axis 3"] items=["Axis 1", "Axis 2", "Axis 3", "Axis 4"] ("Start Axes Select")
                    n102 = call <vilib>:"Single Axis Load Velocity Override.vi"("error in (no error)"=w345, "Override Velosity Value"=w341, "Axis Select"=Axis_Select."Axis 1", "GECO Motion in"=w346) -> ("error out"=w351:errorcluster, "GECO Motion out"=w352:refnum<class "GECO Motion.lvclass">)  [unwired: 5 in, 1 out]
                    n103 = call <vilib>:"Single Axis Load Velocity Override.vi"("error in (no error)"=w351, "Override Velosity Value"=w341, "Axis Select"=Axis_Select."Axis 2", "GECO Motion in"=w352) -> ("error out"=w349:errorcluster, "GECO Motion out"=w350:refnum<class "GECO Motion.lvclass">)  [unwired: 5 in, 1 out]
                    n104 = call <vilib>:"Single Axis Load Velocity Override.vi"("error in (no error)"=w349, "Override Velosity Value"=w341, "Axis Select"=Axis_Select."Axis 3", "GECO Motion in"=w350) -> ("error out"=w347:errorcluster, "GECO Motion out"=w348:refnum<class "GECO Motion.lvclass">)  [unwired: 5 in, 1 out]
                    n105 = call <vilib>:"MultiAxes Sync Move Start.vi"("error in (no error)"=w347, "Start Axes Select"=w342, "GECO Motion in"=w348) -> ("error out"=w353:errorcluster, "GECO Motion out"=w354:refnum<class "GECO Motion.lvclass">)  [unwired: 7 in]
                  }
                }
              }
              frame 7 {
                n106 = Unbundle By Name(w356) -> ("三軸同退"=w355:bool)
                n107 = case shown="False" w355 {
                  tunnel: w361 -> [w365 w385]
                  tunnel: w360 -> [w366 w384]
                  tunnel: w359 -> [_ w378]
                  tunnel: [w363 w393] -> w358
                  tunnel: [w362 w392] -> w357
                  frame False {
                    w364 = T4[] [enum."Axis 1", enum."Axis 2", enum."Axis 3"] items=["Axis 1", "Axis 2", "Axis 3", "Axis 4"] ("Start Axes Select")
                    n108 = for {
                      tunnel: w366 -> [w375]
                      tunnel: w365 -> [w374]
                      tunnel: w364 -> [w373] mode=indexing
                      tunnel: [w368] -> w363
                      tunnel: [w369] -> w362
                      w376 = u16 0 items=["Decelerate", "Halt"] ("Motion Stop Type")
                      n109 = call <vilib>:"Single Axis Move Stop.vi"("error in (no error)"=w375, "Motion Stop Type"=w376, "Axis Select"=w373, "GECO Motion in"=w374) -> ("error out"=w371:errorcluster, "Axis Select out"=w370:T4, "GECO Motion out"=w372:refnum<class "GECO Motion.lvclass">)  [unwired: 5 in]
                      n110 = call <vilib>:"Single Axis Load Velocity Override.vi"("error in (no error)"=w371, "Override Velosity Value"=0, "Axis Select"=w370, "GECO Motion in"=w372) -> ("error out"=w369:errorcluster, "GECO Motion out"=w368:refnum<class "GECO Motion.lvclass">)  [unwired: 5 in, 1 out]
                    }
                  }
                  frame True {
                    w381 = T4[] [enum."Axis 1", enum."Axis 2", enum."Axis 3"] items=["Axis 1", "Axis 2", "Axis 3", "Axis 4"] ("Start Axes Select")
                    n111 = Multiply(x=w378, y=-1) -> (x*y=w379:i32)
                    n112 = call <vilib>:"Single Axis Load Velocity Override.vi"("error in (no error)"=w384, "Override Velosity Value"=w379, "Axis Select"=Axis_Select."Axis 1", "GECO Motion in"=w385) -> ("error out"=w390:errorcluster, "GECO Motion out"=w391:refnum<class "GECO Motion.lvclass">)  [unwired: 5 in, 1 out]
                    n113 = call <vilib>:"Single Axis Load Velocity Override.vi"("error in (no error)"=w390, "Override Velosity Value"=w379, "Axis Select"=Axis_Select."Axis 2", "GECO Motion in"=w391) -> ("error out"=w388:errorcluster, "GECO Motion out"=w389:refnum<class "GECO Motion.lvclass">)  [unwired: 5 in, 1 out]
                    n114 = call <vilib>:"Single Axis Load Velocity Override.vi"("error in (no error)"=w388, "Override Velosity Value"=w379, "Axis Select"=Axis_Select."Axis 3", "GECO Motion in"=w389) -> ("error out"=w386:errorcluster, "GECO Motion out"=w387:refnum<class "GECO Motion.lvclass">)  [unwired: 5 in, 1 out]
                    n115 = call <vilib>:"MultiAxes Sync Move Start.vi"("error in (no error)"=w386, "Start Axes Select"=w381, "GECO Motion in"=w387) -> ("error out"=w392:errorcluster, "GECO Motion out"=w393:refnum<class "GECO Motion.lvclass">)  [unwired: 7 in]
                  }
                }
              }
            }
            n116 = Bundle By Name(cluster=w108, "GECO Motion out"=w109) -> (w114:T3)
          }
          frame "ZABMove" {
            w395 = T4[] [enum."Axis 1", enum."Axis 2", enum."Axis 3"] items=["Axis 1", "Axis 2", "Axis 3", "Axis 4"] ("Start Axes Select")
            n117 = Unbundle By Name(w406) -> ("PIDSetting.Move Setting"=w407:T9, "GECO Motion out"=w396:refnum<class "GECO Motion.lvclass">)
            n118 = call <vilib>:"MultiAxes Sync Move Start.vi"("error in (no error)"=w397, "Start Axes Select"=w395, "GECO Motion in"=w396) -> ("error out"=w398:errorcluster, "GECO Motion out"=w399:refnum<class "GECO Motion.lvclass">)  [unwired: 7 in]
            n119 = case shown="1" w407 {
              selector: w407 -> [_ w422 w529 _ _]
              tunnel: w406 -> [_ w444 w526 w532 w535]
              tunnel: w398 -> [w412 w453 w528 w531 w534]
              tunnel: [w411 w419 w480 w531 w534] -> w405
              tunnel: [w410 w423 w481 w530 w533] -> w403
              tunnel: [_ _ w467 _ _] -> w402
              tunnel: [_ _ w466 _ _] -> w401
              tunnel: [_ _ w465 _ _] -> w400
              tunnel: w399 -> [w408 _ w527 _ _]
              tunnel: [_ _ w468 _ _] -> w394
              frame Default {
                w409 = T4[] [enum."Axis 1", enum."Axis 2", enum."Axis 3", enum."Axis 4"] items=["Axis 1", "Axis 2", "Axis 3", "Axis 4"]
                n120 = for {
                  tunnel: w412 -> [w415]
                  tunnel: [w413] -> w411
                  tunnel: [w414] -> w410
                  tunnel: w409 -> [w417] mode=indexing
                  tunnel: w408 -> [w418]
                  w416 = u16 0 items=["Decelerate", "Halt"] ("Motion Stop Type")
                  n121 = call <vilib>:"Single Axis Move Stop.vi"("error in (no error)"=w415, "Motion Stop Type"=w416, "Axis Select"=w417, "GECO Motion in"=w418) -> ("error out"=w413:errorcluster, "GECO Motion out"=w414:refnum<class "GECO Motion.lvclass">)  [unwired: 5 in, 1 out]
                }
              }
              frame 0 {
                w432 = T4[] [enum."Axis 1", enum."Axis 2", enum."Axis 3"] items=["Axis 1", "Axis 2", "Axis 3", "Axis 4"] ("Start Axes Select")
                # "輸入Z、A、B"
                n122 = Unbundle By Name(w444) -> ("PIDSetting.Z"=w450:i32, "PIDSetting.A"=w449:i32, "PIDSetting.B"=w448:i32, "PIDSetting.Axis Length"=w458:dbl, "PIDSetting.Axis Pulse"=w454:dbl, "GECO Motion out"=w452:refnum<class "GECO Motion.lvclass">)
                n123 = Unbundle By Name(w444) -> ("ServoSetting.Singel Axis Move Paramters.Velocity (10000)"=w427:i32)
                n124 = call "綜合圓軌跡子VI.vi"("Ring"=w422, "移動z"=w450, "al"=w449, "be"=w448) -> ("Z"=w424:dbl, "A"=w425:dbl, "B"=w426:dbl)  [unwired: 2 in]
                n125 = call "推導公式.vi"("be"=w426, "al"=w425, "移動z"=w424) -> ("L3"=w459:dbl, "L2"=w460:dbl, "L1"=w461:dbl)
                n126 = Subtract(x=w461, y=w458) -> (x-y=w457:dbl)
                n127 = Subtract(x=w460, y=w458) -> (x-y=w456:dbl)
                n128 = Subtract(x=w459, y=w458) -> (x-y=w455:dbl)
                n129 = Multiply(x=w457, y=w454) -> (x*y=w420:dbl)
                n130 = Multiply(x=w456, y=w454) -> (x*y=w429:dbl)
                n131 = Multiply(x=w455, y=w454) -> (x*y=w421:dbl)
                n132 = call <vilib>:"Single Axis Load Velocity Override.vi"("error in (no error)"=w453, "Override Velosity Value"=w427, "Axis Select"=Axis_Select."Axis 1" ("Single Axis Select"), "GECO Motion in"=w452) -> ("error out"=w446:errorcluster, "Axis Select out"=w445:T4, "GECO Motion out"=w447:refnum<class "GECO Motion.lvclass">)  [unwired: 5 in]
                n133 = call <vilib>:"Single Axis Load Position Override.vi"("error in (no error)"=w446, "Override Target Position Value"=w421, "Axis Select"=w445, "GECO Motion in"=w447) -> ("error out"=w442:errorcluster, "GECO Motion out"=w443:refnum<class "GECO Motion.lvclass">)  [unwired: 5 in, 1 out]
                n134 = call <vilib>:"Single Axis Load Velocity Override.vi"("error in (no error)"=w442, "Override Velosity Value"=w427, "Axis Select"=Axis_Select."Axis 2" ("Single Axis Select"), "GECO Motion in"=w443) -> ("error out"=w439:errorcluster, "Axis Select out"=w438:T4, "GECO Motion out"=w440:refnum<class "GECO Motion.lvclass">)  [unwired: 5 in]
                n135 = call <vilib>:"Single Axis Load Position Override.vi"("error in (no error)"=w439, "Override Target Position Value"=w429, "Axis Select"=w438, "GECO Motion in"=w440) -> ("error out"=w433:errorcluster, "GECO Motion out"=w434:refnum<class "GECO Motion.lvclass">)  [unwired: 5 in, 1 out]
                n136 = call <vilib>:"Single Axis Load Velocity Override.vi"("error in (no error)"=w433, "Override Velosity Value"=w427, "Axis Select"=Axis_Select."Axis 3" ("Single Axis Select"), "GECO Motion in"=w434) -> ("error out"=w436:errorcluster, "Axis Select out"=w435:T4, "GECO Motion out"=w437:refnum<class "GECO Motion.lvclass">)  [unwired: 5 in]
                n137 = call <vilib>:"Single Axis Load Position Override.vi"("error in (no error)"=w436, "Override Target Position Value"=w420, "Axis Select"=w435, "GECO Motion in"=w437) -> ("error out"=w430:errorcluster, "GECO Motion out"=w431:refnum<class "GECO Motion.lvclass">)  [unwired: 5 in, 1 out]
                n138 = call <vilib>:"MultiAxes Sync Move Start.vi"("error in (no error)"=w430, "Start Axes Select"=w432, "GECO Motion in"=w431) -> ("error out"=w419:errorcluster, "GECO Motion out"=w423:refnum<class "GECO Motion.lvclass">)  [unwired: 7 in]
              }
              frame 1 {
                w525 = cluster{"output high":dbl, "output low":dbl} {"output high"=200000.0, "output low"=-500000.0} ("PID Def Output range")
                w493 = Axis_Select."Axis 3" ("Single Axis Select")
                w494 = Axis_Select."Axis 2" ("Single Axis Select")
                w492 = Axis_Select."Axis 1" ("Single Axis Select")
                # "PID取樣時間"
                # "Stm32 Delay Time"
                # "圓軌跡"
                n139 = Unbundle By Name(w526) -> ("PIDSetting.Axis Length"=w501:dbl, "PIDSetting.Axis Pulse"=w515:dbl)
                n140 = feedback #1() -> (w472:i32)
                n141 = Increment(x=w472) -> (x+1=w473:i32)
                n142 = feedback-in #1(w473) -> ()
                n143 = call <vilib>:"Read Encoder Position.vi"("error in (no error)"=w528, "Axis Select"=w492, "GECO Motion in"=w527) -> ("error out"=w499:errorcluster, "GECO Motion out"=w500:refnum<class "GECO Motion.lvclass">, "Encoder Position"=w479:i32, "Logical Position"=w491:i32)  [unwired: 4 in, 1 out]
                n144 = call <vilib>:"Read Encoder Position.vi"("error in (no error)"=w499, "Axis Select"=w494, "GECO Motion in"=w500) -> ("error out"=w497:errorcluster, "GECO Motion out"=w498:refnum<class "GECO Motion.lvclass">, "Encoder Position"=w478:i32, "Logical Position"=w490:i32)  [unwired: 4 in, 1 out]
                n145 = Bundle("Encoder Position"=w479, "Logical Position"=w491) -> (w467:T1)  [unwired: 1 in]
                n146 = call <vilib>:"Read Encoder Position.vi"("error in (no error)"=w497, "Axis Select"=w493, "GECO Motion in"=w498) -> ("error out"=w495:errorcluster, "GECO Motion out"=w496:refnum<class "GECO Motion.lvclass">, "Encoder Position"=w477:i32, "Logical Position"=w489:i32)  [unwired: 4 in, 1 out]
                n147 = call "綜合圓軌跡子VI.vi"("Ring"=w529, "I時間"=w472) -> ("Z"=w522:dbl, "A"=w471:dbl, "B"=w470:dbl)  [unwired: 4 in]
                n148 = property on="Axis 1" class="Clust (strict)"("Value"=w467) -> ()  [unwired: 2 in, 2 out]
                n149 = call "推導公式.vi"("be"=w470, "al"=w471, "移動z"=w522) -> ("L3"=w516:dbl, "L2"=w517:dbl, "L1"=w518:dbl)
                n150 = shared-variable "My Computer\\PC_Variables.lvlib\\PID gains"() -> (w464:T20)  [unwired: 1 in, 1 out]
                n151 = shared-variable "My Computer\\PC_Variables.lvlib\\PID gains 2"() -> (w463:T20)  [unwired: 1 in, 1 out]
                n152 = shared-variable "My Computer\\PC_Variables.lvlib\\PID gains 3"() -> (w462:T20)  [unwired: 1 in, 1 out]
                n153 = Bundle("Encoder Position"=w478, "Logical Position"=w490) -> (w466:T1)  [unwired: 1 in]
                n154 = Subtract(x=w518, y=w501) -> (x-y=w521:dbl)
                n155 = Subtract(x=w517, y=w501) -> (x-y=w520:dbl)
                n156 = Subtract(x=w516, y=w501) -> (x-y=w519:dbl)
                n157 = property on="Axis 2" class="Clust (strict)"("Value"=w466) -> ()  [unwired: 2 in, 2 out]
                n158 = feedback #2() -> (w476:i32)
                n159 = feedback-in #2(w479) -> ()
                n160 = feedback #3() -> (w475:i32)
                n161 = feedback-in #3(w478) -> ()
                n162 = feedback #4() -> (w474:i32)
                n163 = feedback-in #4(w477) -> ()
                n164 = Multiply ("L1 pulse")(x=w521, y=w515) -> (x*y=w487:dbl)
                n165 = Multiply ("L2 pulse")(x=w520, y=w515) -> (x*y=w486:dbl)
                n166 = Multiply ("L3 pulse")(x=w519, y=w515) -> (x*y=w485:dbl)
                n167 = Divide(x=25.0, y=1000.0) -> (x/y=w514:dbl)
                n168 = Bundle("Encoder Position"=w477, "Logical Position"=w489) -> (w465:T1)  [unwired: 1 in]
                n169 = property on="Axis 3" class="Clust (strict)"("Value"=w465) -> ()  [unwired: 2 in, 2 out]
                n170 = call-poly <vilib>:"PID.vi"("output range"=w525, "dt (s)"=w514, "PID gains"=w464, "process variable"=w476, "setpoint"=w485) -> ("output"=w484:dbl)  [unwired: 5 in, 1 out]
                n171 = call-poly <vilib>:"PID.vi"("output range"=w525, "dt (s)"=w514, "PID gains"=w463, "process variable"=w475, "setpoint"=w486) -> ("output"=w483:dbl)  [unwired: 5 in, 1 out]
                n172 = call-poly <vilib>:"PID.vi"("output range"=w525, "dt (s)"=w514, "PID gains"=w462, "process variable"=w474, "setpoint"=w487) -> ("output"=w482:dbl)  [unwired: 5 in, 1 out]
                n173 = call <vilib>:"Single Axis Load Velocity Override.vi"("error in (no error)"=w495, "Override Velosity Value"=w484, "Axis Select"=w492, "GECO Motion in"=w496) -> ("error out"=w512:errorcluster, "Axis Select out"=w504:T4, "GECO Motion out"=w513:refnum<class "GECO Motion.lvclass">)  [unwired: 5 in]
                n174 = call <vilib>:"Single Axis Load Position Override.vi"("error in (no error)"=w512, "Axis Select"=w504, "GECO Motion in"=w513) -> ("error out"=w510:errorcluster, "GECO Motion out"=w511:refnum<class "GECO Motion.lvclass">)  [unwired: 6 in, 1 out]
                n175 = shared-variable "My Computer\\PC_Variables.lvlib\\Axis 1 Position"(w467) -> ()  [unwired: 1 in, 1 out]
                n176 = call <vilib>:"Single Axis Load Velocity Override.vi"("error in (no error)"=w510, "Override Velosity Value"=w483, "Axis Select"=w494, "GECO Motion in"=w511) -> ("error out"=w488:errorcluster, "Axis Select out"=w503:T4, "GECO Motion out"=w509:refnum<class "GECO Motion.lvclass">)  [unwired: 5 in]
                n177 = call <vilib>:"Single Axis Load Position Override.vi"("error in (no error)"=w488, "Axis Select"=w503, "GECO Motion in"=w509) -> ("error out"=w507:errorcluster, "GECO Motion out"=w508:refnum<class "GECO Motion.lvclass">)  [unwired: 6 in, 1 out]
                n178 = call <vilib>:"Single Axis Load Velocity Override.vi"("error in (no error)"=w507, "Override Velosity Value"=w482, "Axis Select"=w493, "GECO Motion in"=w508) -> ("error out"=w505:errorcluster, "Axis Select out"=w502:T4, "GECO Motion out"=w506:refnum<class "GECO Motion.lvclass">)  [unwired: 5 in]
                n179 = shared-variable "My Computer\\PC_Variables.lvlib\\Axis 2 Position"(w466) -> ()  [unwired: 1 in, 1 out]
                n180 = call <vilib>:"Single Axis Load Position Override.vi"("error in (no error)"=w505, "Axis Select"=w502, "GECO Motion in"=w506) -> ("error out"=w480:errorcluster, "GECO Motion out"=w481:refnum<class "GECO Motion.lvclass">)  [unwired: 6 in, 1 out]
                n181 = shared-variable "My Computer\\PC_Variables.lvlib\\Axis 3 Position"(w465) -> ()  [unwired: 1 in, 1 out]
                n182 = Bundle By Name(cluster=cluster{"A":dbl, "B":dbl} {"A"=0.0, "B"=0.0} ("理想角度"), "A"=w471, "B"=w470) -> (w468:cluster{"A":dbl, "B":dbl})
              }
              frame 2 {
                # "Á³±Û­y¸ñ"
                n183 = Unbundle By Name(w532) -> ("GECO Motion out"=w530:refnum<class "GECO Motion.lvclass">)
              }
              frame 3 {
                # "Z上下"
                n184 = Unbundle By Name(w535) -> ("GECO Motion out"=w533:refnum<class "GECO Motion.lvclass">)
              }
            }
            n185 = Bundle By Name(cluster=w406, "GECO Motion out"=w403, "Axis 1 Position"=w402, "Axis 2 Position"=w401, "Axis 3 Position"=w400, "理想角度"=w394) -> (w404:T3)
          }
          frame "AlarmReset" {
            w542 = T4[] [enum."Axis 1", enum."Axis 2", enum."Axis 3", enum."Axis 4"] items=["Axis 1", "Axis 2", "Axis 3", "Axis 4"]
            n186 = Unbundle By Name(w541) -> ("GECO Motion out"=w539:refnum<class "GECO Motion.lvclass">)
            n187 = for {
              tunnel: [w551] -> w537
              tunnel: [w550] -> w536
              tunnel: w542 -> [w545] mode=indexing
              tunnel: w540 -> [w547]
              tunnel: w539 -> [w546]
              w543 = u16 0 items=["Decelerate", "Halt"] ("Motion Stop Type")
              n188 = call <vilib>:"Single Axis Move Stop.vi"("error in (no error)"=w547, "Motion Stop Type"=w543, "Axis Select"=w545, "GECO Motion in"=w546) -> ("error out"=w548:errorcluster, "Axis Select out"=w544:T4, "GECO Motion out"=w549:refnum<class "GECO Motion.lvclass">)  [unwired: 5 in]
              n189 = call <vilib>:"Alarm Reset.vi"("error in (no error)"=w548, "Axis Select"=w544, "GECO Motion in"=w549) -> ("error out"=w550:errorcluster, "GECO Motion out"=w551:refnum<class "GECO Motion.lvclass">)  [unwired: 6 in, 1 out]
            }
            n190 = Bundle By Name(cluster=w541, "GECO Motion out"=w537) -> (w538:T3)
          }
          frame "EncoderReset" {
            w558 = T4[] [enum."Axis 1", enum."Axis 2", enum."Axis 3", enum."Axis 4"] items=["Axis 1", "Axis 2", "Axis 3", "Axis 4"]
            n191 = Unbundle By Name(w557) -> ("GECO Motion out"=w555:refnum<class "GECO Motion.lvclass">)
            n192 = for {
              tunnel: [w567] -> w553
              tunnel: [w566] -> w552
              tunnel: w558 -> [w565] mode=indexing
              tunnel: w556 -> [w562]
              tunnel: w555 -> [w561]
              w559 = u16 0 items=["Decelerate", "Halt"] ("Motion Stop Type")
              n193 = call <vilib>:"Single Axis Move Stop.vi"("error in (no error)"=w562, "Motion Stop Type"=w559, "Axis Select"=w565, "GECO Motion in"=w561) -> ("error out"=w563:errorcluster, "Axis Select out"=w560:T4, "GECO Motion out"=w564:refnum<class "GECO Motion.lvclass">)  [unwired: 5 in]
              n194 = call <vilib>:"Reset Encoder Position.vi"("error in (no error)"=w563, "Axis Select"=w560, "GECO Motion in"=w564) -> ("error out"=w566:errorcluster, "GECO Motion out"=w567:refnum<class "GECO Motion.lvclass">)  [unwired: 6 in, 1 out]
            }
            n195 = Bundle By Name(cluster=w557, "GECO Motion out"=w553) -> (w554:T3)
          }
          frame "LinkBoard" {
            n196 = Unbundle By Name(w588) -> ("resource name"=w578:tag, "TCP slave port"=w586:u16, "ServoSetting.Motion Controller Slot"=w579:T7)
            n197 = Format Date/Time String(time format string (%c)="%Y %m %d %H %M ") -> (date/time string=w575:string)  [unwired: 2 in]
            n198 = Concatenate Strings(w575, "Ideal Angle.txt" ("element")) -> (w574:string)
            n199 = Build Path(base path=path "u:/data", name or relative path=w574) -> (appended path=w576:path)
            n200 = Open/Create/Replace File(file path (use dialog)=w576, error in=w570, operation (0:open)=T16."replace or create") -> (refnum out=w568:refnum<file>, error out=w571:errorcluster)  [unwired: 3 in, 1 out]
            n201 = call-poly <vilib>:"Create Modbus Instance.vi"("error in"=w571, "port (502)"=w586) -> ("error out"=w585:errorcluster, "TCP slave instance"=w580:refnum<class "Modbus Slave.lvclass">)  [unwired: 8 in]
            n202 = call-poly <vilib>:"Initialize.vi"("error in (no error)"=w585, "resource name"=w578) -> ("error out"=w584:errorcluster, "GECO_Driver out"=w581:refnum<class "GECO_Driver.lvclass">)  [unwired: 8 in]
            n203 = call <vilib>:"Initialize Motion Controller.vi"("error in (no error)"=w584, "Slot"=w579, "GECO_Driver in"=w581) -> ("error out"=w582:errorcluster, "Motion reference out"=w583:refnum<class "GECO Motion.lvclass">)  [unwired: 7 in]
            n204 = Bundle By Name(cluster=w588, "Modbus COM"=w580, "GECO_Driver out"=w581, "GECO Motion out"=w583, "Save Path"=w568) -> (w587:T3)
          }
          frame "PanelUpdate" {
            n205 = Unbundle By Name(w611) -> ("GECO Motion out"=w610:refnum<class "GECO Motion.lvclass">)
            n206 = call <vilib>:"Read Encoder Position.vi"("error in (no error)"=w613, "Axis Select"=Axis_Select."Axis 1", "GECO Motion in"=w610) -> ("error out"=w606:errorcluster, "GECO Motion out"=w607:refnum<class "GECO Motion.lvclass">, "Encoder Position"=w599:i32, "Logical Position"=w600:i32)  [unwired: 4 in, 1 out]
            n207 = Bundle(cluster=T17 {"Logical Position"=0, "Encoder Position"=0} ("input cluster"), "Logical Position"=w600, "Encoder Position"=w599) -> (w591:T17)
            "Axis 1" <- w591
            n208 = shared-variable "My Computer\\PC_Variables.lvlib\\Axis 1 Position"(w591) -> ()  [unwired: 1 in, 1 out]
            n209 = call <vilib>:"Read Encoder Position.vi"("error in (no error)"=w606, "Axis Select"=Axis_Select."Axis 2", "GECO Motion in"=w607) -> ("error out"=w604:errorcluster, "GECO Motion out"=w605:refnum<class "GECO Motion.lvclass">, "Encoder Position"=w592:i32, "Logical Position"=w593:i32)  [unwired: 4 in, 1 out]
            n210 = Bundle(cluster=T17 {"Logical Position"=0, "Encoder Position"=0} ("input cluster"), "Logical Position"=w593, "Encoder Position"=w592) -> (w590:T17)
            "Axis 2" <- w590
            n211 = shared-variable "My Computer\\PC_Variables.lvlib\\Axis 2 Position"(w590) -> ()  [unwired: 1 in, 1 out]
            n212 = call <vilib>:"Read Encoder Position.vi"("error in (no error)"=w604, "Axis Select"=Axis_Select."Axis 3", "GECO Motion in"=w605) -> ("error out"=w612:errorcluster, "GECO Motion out"=w608:refnum<class "GECO Motion.lvclass">, "Encoder Position"=w594:i32, "Logical Position"=w595:i32)  [unwired: 4 in, 1 out]
            n213 = Bundle(cluster=T17 {"Logical Position"=0, "Encoder Position"=0} ("input cluster"), "Logical Position"=w595, "Encoder Position"=w594) -> (w589:T17)
            "Axis 3" <- w589
            n214 = shared-variable "My Computer\\PC_Variables.lvlib\\Axis 3 Position"(w589) -> ()  [unwired: 1 in, 1 out]
            n215 = Bundle By Name(cluster=w611, "GECO Motion out"=w608, "Axis 1 Position"=w591, "Axis 2 Position"=w590, "Axis 3 Position"=w589) -> (w609:T3)
          }
          frame "CloseBoard" {
            w614 = T4[] [enum."Axis 1", enum."Axis 2", enum."Axis 3", enum."Axis 4"] items=["Axis 1", "Axis 2", "Axis 3", "Axis 4"]
            n216 = Unbundle By Name(w620) -> ("GECO_Driver out"=w616:refnum<class "GECO_Driver.lvclass">, "GECO Motion out"=w615:refnum<class "GECO Motion.lvclass">)
            n217 = for {
              tunnel: [w625] -> w617
              tunnel: w615 -> [w624]
              tunnel: w618 -> [w623]
              tunnel: w614 -> [w621] mode=indexing
              n218 = call <vilib>:"Servo On.vi"("error in (no error)"=w623, "Servo On"=FALSE, "Axis Select"=w621, "GECO Motion in"=w624) -> ("error out"=w628:errorcluster, "Axis Select out"=w627:T4, "GECO Motion out"=w626:refnum<class "GECO Motion.lvclass">)  [unwired: 5 in]
              n219 = call <vilib>:"Single Axis Move Stop.vi"("error in (no error)"=w628, "Axis Select"=w627, "GECO Motion in"=w626) -> ("error out"=w625:errorcluster)  [unwired: 6 in, 2 out]
            }
            n220 = call <vilib>:"Close.vi"("error in (no error)"=w617, "GECO_Driver in"=w616) -> ("error out"=w619:errorcluster)  [unwired: 9 in]
          }
        }
        n221 = Unbundle By Name(w21) -> ("status"=w22:bool)
      }
      frame Error {
      }
    }
    n222 = Tick Count (ms)() -> (millisecond timer value=w16:u32)
    n223 = Unbundle By Name(w14) -> ("理想角度"=w13:cluster{"A":dbl, "B":dbl})
    n224 = Subtract(x=w16, y=w15) -> (x-y=w12:u32)
    "Program Period" <- w12
    n225 = shared-variable "NI-sbRIO9606-01F1BAB2\\RT_Variables.lvlib\\Program Period"(w12) -> ()  [unwired: 1 in, 1 out]
  }
  n226 = Unbundle By Name(w3) -> ("Save Path"=w2:refnum<file>)
  n227 = for {
    tunnel: [w641] -> w1 mode=indexing
    tunnel: w5 -> [w640] mode=indexing
    tunnel: w4 -> [w637] mode=indexing
    n228 = Unbundle(w640) -> ("A"=w639:dbl, "B"=w638:dbl)
    n229 = Format Into String(w639) -> (resulting string=w634:string)  [unwired: 3 in, 1 out]
    n230 = Format Into String(w638) -> (resulting string=w632:string)  [unwired: 3 in, 1 out]
    n231 = Format Into String(w637) -> (resulting string=w636:string)  [unwired: 3 in, 1 out]
    n232 = Insert Into Array(array=string[] ["Program Period(ms)："], new element #1=w636, new element #2="A：", new element #3=w634, new element #4="B：", new element #5=w632) -> (w641:string[])  [unwired: 1 in]
  }
  n233 = for {
    tunnel: w1 -> [w645] mode=indexing
    shift-right: [w643] -> _
    shift-left: w2 -> [w647]
    shift-right: [w644] -> _
    shift-left: _ -> [w646]
    n234 = Array To Spreadsheet String(delimiter (Tab)="\t", array=w645, 3:"%f" ("format string")) -> (spreadsheet string=w648:string)
    n235 = Write to Text File(file (use dialog)=w647, text=w648, error in=w646) -> (refnum out=w643:refnum<file>, error out=w644:errorcluster)  [unwired: 1 in, 1 out]
  }
